vi "Write Config info.vi"(10 "Config info":T1={"Frequency (MHz)"="", "Power (dBm)"="", "Loop order"=enum."Device -> Power -> Frequency", "SG loss"=TRUE, "PM loss"=TRUE, "SG"=1}, 11 "RF Power in":refnum<class "RF Power.lvclass">) -> (3 "RF Power out":refnum<class "RF Power.lvclass">)   [LabVIEW 2020, in "RF Power.lvclass"]
uses:
  RF Power.lvclass
  Controls/Config info.ctl
  Controls/Loop order.ctl
  RF Power.lvclass/RF Power.ctl
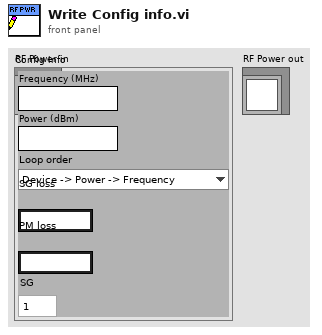
[diagram p1: front panel]
types:
  T1 = typedef "RF Power.lvclass/Config info.ctl" = cluster{"Frequency (MHz)":string, "Power (dBm)":string, "Loop order":T2, "SG loss":bool, "PM loss":bool, "SG":i32}
  T2 = typedef "RF Power.lvclass/Loop order.ctl" = enum16{"Device -> Power -> Frequency", "Device -> Frequency -> Power"}
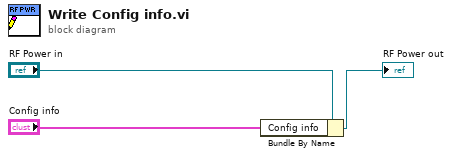
[diagram p0: block diagram]
diagram:
  n1 = Bundle By Name(cluster="RF Power in", "Config info"="Config info") -> (→"RF Power out":refnum<class "RF Power.lvclass">)
